vi "SetWindowSize.vi"(8 "No Error":errorcluster, 9 "h":i32, 10 "w":i32, 11 "window [SDL_Window *]":i64) -> (0 "error out":errorcluster)   [LabVIEW 2024, in "SDL3.lvlib" / "Video.lvlib"]
doc: "Request that the size of a window's client area be set."
uses:
  Video.lvlib
  Error/Error.lvlib
  _LV-SDL3/Lib/SDL3-32.dll
panel:
  # "https://wiki.libsdl.org/SDL3/SDL_SetWindowSize"
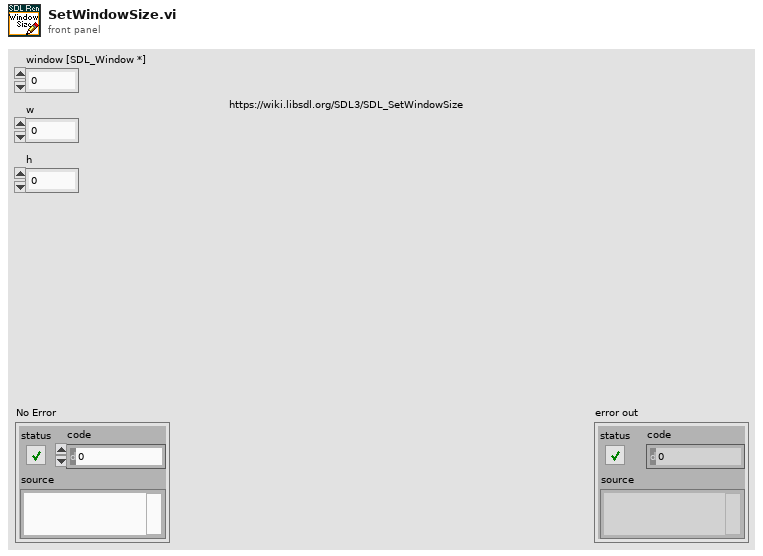
[diagram p1: front panel]
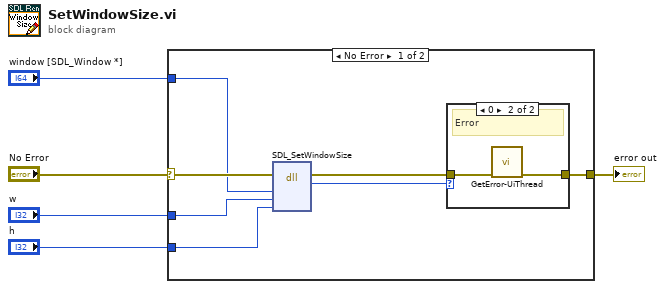
[diagram p0: block diagram]
diagram:
  n1 = case shown="No Error" "No Error" {
    selector: "No Error" -> [w12 w16]
    tunnel: [w10 w16] -> w4
    tunnel: "w" -> [w8 _]
    tunnel: "h" -> [w7 _]
    tunnel: "window [SDL_Window *]" -> [w6 _]
    frame No Error {
      n2 = dll-call lib="C:/Users/Thomas/Documents/Projects/_LV-SDL3/Lib/SDL3-*.*" fn="SDL_SetWindowSize"(error in=w12, "window"=w6, "w"=w8, "h"=w7) -> (error out=w11:errorcluster, "return type"=w9:i64)  [unwired: 5 in, 1 out]
      n3 = case shown="0" w9 {
        tunnel: w11 -> [w13 w15]
        tunnel: [w13 w14] -> w10
        frame Default {
          # "Ok"
        }
        frame 0 {
          # "Error"
          n4 = call "GetError-UiThread.vi"("No Error"=w15) -> ("error out"=w14:errorcluster)  [unwired: 10 in]
        }
      }
    }
    frame Error {
    }
  }
  "error out" <- w4
